vi "Remove State Callback.vi"(7 "Owner":refnum<class>, 8 "error in (no error)":errorcluster, 10 "Callback":refnum<vi>, 11 "Endpoint in":refnum<class "Endpoint.lvclass">) -> (0 "error out":errorcluster, 2 "Found":bool, 3 "Endpoint out":refnum<class "Endpoint.lvclass">)   [LabVIEW 2020, in "Stream.lvlib" / "Endpoint.lvclass"]
uses:
  Endpoint.lvclass
  Connection/Connection.lvclass
  State Callback.ctl
  Endpoint.lvclass/Endpoint.ctl
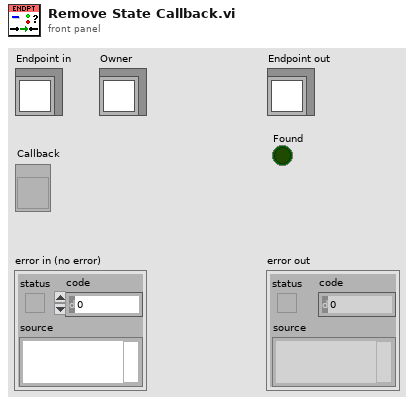
[diagram p1: front panel]
types:
  T1 = typedef "Stream.lvlib/Endpoint.lvclass/State Callback.ctl" = cluster{"Owner":refnum<class>, "VI":refnum<vi>}
  T2 = typedef "Stream.lvlib/Endpoint.lvclass/Ref Data.ctl" = cluster{"URI":refnum<class "URI.lvclass">, "State Callbacks":T1[]}
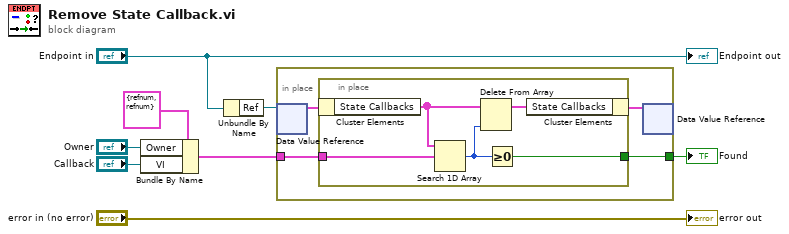
[diagram p0: block diagram]
diagram:
  n1 = Bundle By Name(cluster=T1 {"Owner"=refnum, "VI"=refnum} ("State Callback"), "Owner"="Owner", "VI"="Callback") -> (w2:T1)
  n2 = Unbundle By Name("Endpoint in") -> ("Ref"=w4:refnum<data-value>)
  n3 = in-place {
    in-place-border: w2 -> [w10]
    in-place-border: [w9] -> w1
    n4 = in-place-dvr #1(w4) -> (w12:T2)  [unwired: 1 out]
    n5 = in-place {
      in-place-border: w10 -> [w17]
      in-place-border: [w13] -> w9
      n6 = in-place-cluster #2(w12) -> ("State Callbacks"=w16:T1[])
      n7 = Search 1D Array(1D array=w16, element=w17) -> (index of element=w14:i32)  [unwired: 1 in]
      n8 = Delete From Array(array=w16, index=w14) -> (array with subset deleted=w15:T1[])  [unwired: 1 in, 1 out]
      n9 = Greater Or Equal To 0?(x=w14) -> (x >= 0?=w13:bool)
      n10 = in-place-cluster #2("State Callbacks"=w15) -> (w11:T2)
    }
    n11 = in-place-dvr #1(w11) -> ()  [unwired: 2 out]
  }
  "Found" <- w1
  "error out" <- "error in (no error)"
  "Endpoint out" <- "Endpoint in"
